vi "Synthetic_jet_global.vi"() -> ()   [LabVIEW 2011]
uses:
  Controls/SJ_Data_Cluster.ctl
panel:
  out "Current Amplitude":dbl
  out "Current Frequency":dbl
  out "Meas Number":i32
  in  "Frequency Array":dbl[](array[numeric])
  in  "SJ Data":T1={"Do (mm)"=3.0, "Dc (mm)"=0.039, "Ho (mm)"=0.01, "Hc (mm)"=0.006, "K"=1.251, "beta"=1.039, "Vc (m^3)"=0.0, "Vo (m^3)"=0.0}
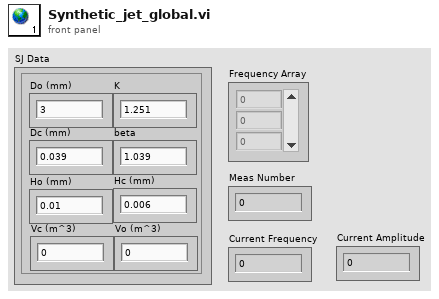
[diagram p1: front panel]
types:
  T1 = typedef "SJ_Data_Cluster.ctl" = cluster{"Do (mm)":dbl, "Dc (mm)":dbl, "Ho (mm)":dbl, "Hc (mm)":dbl, "K":dbl, "beta":dbl, "Vc (m^3)":dbl, "Vo (m^3)":dbl}
diagram:
